vi "Enqueue Error.vi"(9 "error in":errorcluster) -> (1 "error out":errorcluster, 3 "Queue out":refnum<queue>)   [LabVIEW 2018]
doc: "Recoge un error en el cable de error y lo inserta en una cola de errores.\n\nEste VI se utiliza en conjunto con el VI \"Escribir error en Log\" para registrar los errores recogidos por todos los VI \"Enqueue error\" repartidos en el software.\n\nEstos VI utilizan variables globales compartidas para referenciar el queue entre ellos"
uses:
  Global/Error Queue Reference.vi
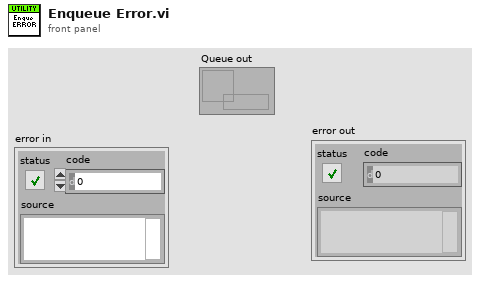
[diagram p1: front panel]
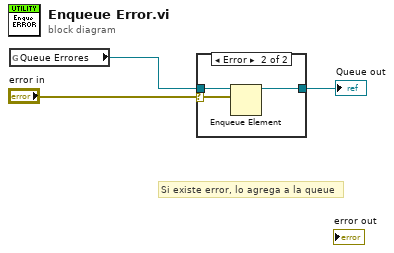
[diagram p0: block diagram]
diagram:
  # "Si existe error, lo agrega a la queue"
  n1 = global read "Error Queue Reference.vi" "Queue Errores"() -> (w2:refnum<queue>)
  n2 = case shown="Error" "error in" {
    selector: "error in" -> [_ w6]
    tunnel: w2 -> [w4 w7]
    tunnel: [w4 w5] -> w3
    frame No Error {
    }
    frame Error {
      n3 = Enqueue Element(queue=w7, element=w6) -> (queue out=w5:refnum<queue>)  [unwired: 2 in, 2 out]
    }
  }
  "Queue out" <- w3
